vi "Build Full Item List.vi"(11 "Components":T2[](array[typedef])) -> (3 "Total Ingredients":T1[](array[typedef]))   [LabVIEW 2020, in "App.lvclass"]
uses:
  App.lvclass
  Blueprint Qty.ctl
  Blueprint/Blueprint.lvclass
  C:/dev/LabVIEW/Good Company Calc/Item/Item.lvclass
  Item/Ingredient.ctl
  Item/Item.lvclass
  Item Batch.ctl
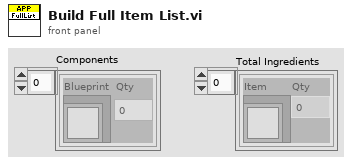
[diagram p1: front panel]
types:
  T1 = typedef "Item.lvclass/Ingredient.ctl" = cluster{"Item":refnum<class "Item.lvclass">, "Qty":dbl}
  T2 = typedef "App.lvclass/Blueprint Qty.ctl" = cluster{"Blueprint":refnum<class "Blueprint.lvclass">, "Qty":dbl}
  T3 = typedef "App.lvclass/Item Batch.ctl" = cluster{"Qty Needed":dbl, "Qty per Batch":dbl, "Batches":dbl}
  T4 = typedef "Item.lvclass/Craft Station.ctl" = cluster{"Station":refnum<class "Workstation.lvclass">, "Craft Time":dbl, "Qty Made":dbl}
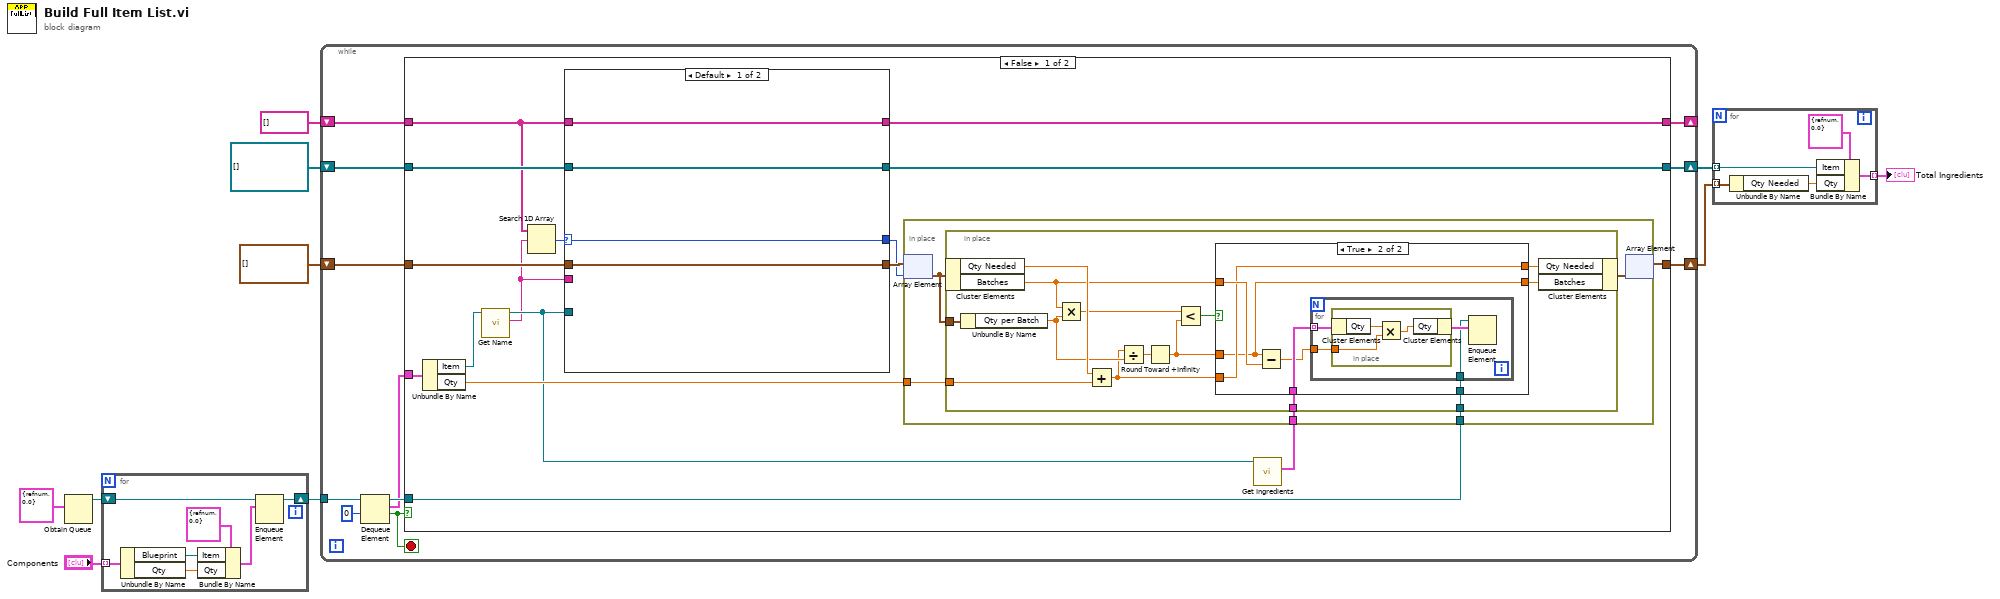
[diagram p0: block diagram]
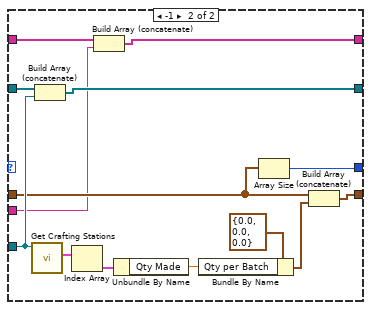
[diagram p2: hidden frame]
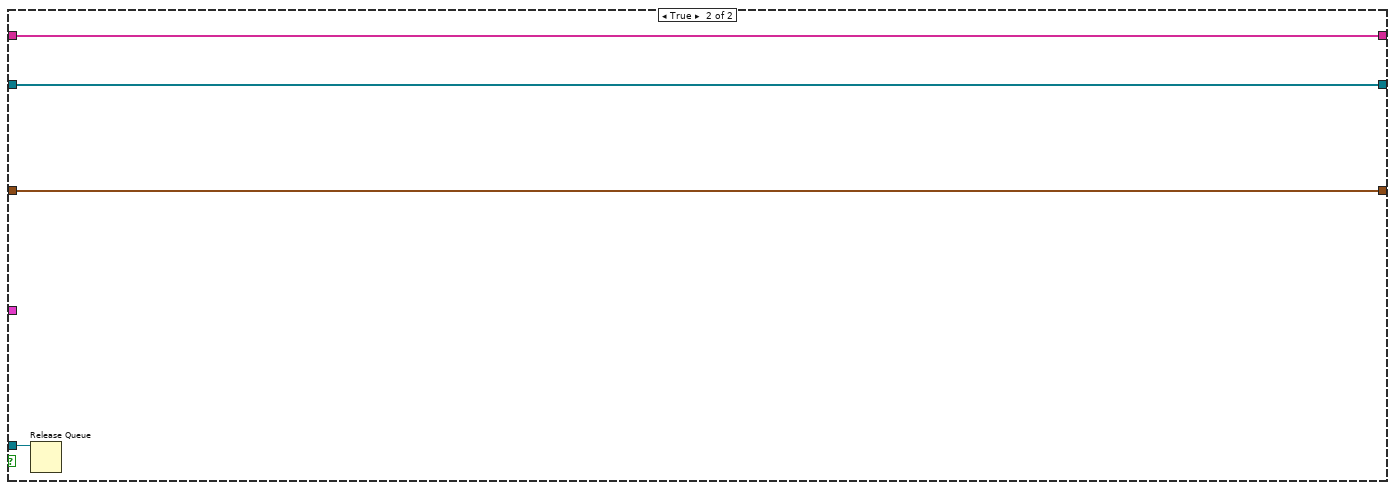
[diagram p4: hidden frame]
diagram:
  n1 = Obtain Queue(element data type=T1 {"Item"=refnum, "Qty"=0.0} ("Ingredient")) -> (queue out=w9:refnum<queue>)  [unwired: 4 in, 2 out]
  n2 = for {
    shift-right: [w16] -> w7
    shift-left: w9 -> [w17]
    tunnel: "Components" -> [w15] mode=indexing
    n3 = Unbundle By Name(w15) -> ("Blueprint"=w13:refnum<class "Blueprint.lvclass">, "Qty"=w12:dbl)
    n4 = Bundle By Name(cluster=T1 {"Item"=refnum, "Qty"=0.0} ("Ingredient"), "Item"=w13, "Qty"=w12) -> (w11:T1)
    n5 = Enqueue Element(queue=w17, element=w11) -> (queue out=w16:refnum<queue>)  [unwired: 2 in, 2 out]
  }
  n6 = while {
    shift-right: [w20] -> w2
    shift-left: T3[] [] -> [w21]
    shift-right: [w22] -> w4
    shift-left: refnum<class "Item.lvclass">[] [] -> [w23]
    tunnel: w7 -> [w28]
    shift-right: [w18] -> _
    shift-left: string[] [] -> [w19]
    stop <- w26 stop-if-true
    n7 = Dequeue Element(queue=w28, timeout in ms (-1)=0) -> (queue out=w25:refnum<queue>, element=w24:T1, timed out?=w26:bool)  [unwired: 1 in, 1 out]
    n8 = case shown="False" w26 {
      tunnel: w25 -> [w39 w99]
      tunnel: w24 -> [w44 _]
      tunnel: w23 -> [w37 w100]
      tunnel: [w43 w100] -> w22
      tunnel: w21 -> [w36 w98]
      tunnel: [w42 w98] -> w20
      tunnel: w19 -> [w32 w97]
      tunnel: [w29 w97] -> w18
      frame False {
        n9 = Unbundle By Name(w44) -> ("Item"=w33:refnum<class "Item.lvclass">, "Qty"=w41:dbl)
        n10 = call-dynamic "Get Name.vi"("Item in"=w33) -> ("Name"=w30:string, "Item out"=w31:refnum<class "Item.lvclass">)  [unwired: 8 in, 1 out]
        n11 = Search 1D Array(1D array=w32, element=w30) -> (index of element=w38:i32)  [unwired: 1 in]
        n12 = case shown="Default" w38 {
          selector: w38 -> [w46 _]
          tunnel: w37 -> [w48 w56]
          tunnel: w31 -> [_ w55]
          tunnel: w36 -> [w47 w53]
          tunnel: [w48 w54] -> w43
          tunnel: [w47 w57] -> w35
          tunnel: [w46 w52] -> w34
          tunnel: w32 -> [w45 w51]
          tunnel: w30 -> [_ w50]
          tunnel: [w45 w49] -> w29
          frame Default {
          }
          frame -1 {
            n13 = call-dynamic "Get Crafting Stations.vi"("Item in"=w55) -> ("Stations"=w62:T4[])  [unwired: 8 in, 2 out]
            n14 = Build Array (concatenate)(w56, w55) -> (w54:refnum<class "Item.lvclass">[])
            n15 = Index Array(array=w62) -> (element=w61:T4)  [unwired: 1 in]
            n16 = Build Array (concatenate)(w51, w50) -> (w49:string[])
            n17 = Unbundle By Name(w61) -> ("Qty Made"=w59:dbl)
            n18 = Bundle By Name(cluster=T3 {"Qty Needed"=0.0, "Qty per Batch"=0.0, "Batches"=0.0} ("Item Batch"), "Qty per Batch"=w59) -> (w58:T3)
            n19 = Array Size(array=w53) -> (size(s)=w52:i32)
            n20 = Build Array (concatenate)(w53, w58) -> (w57:T3[])
          }
        }
        n21 = call-dynamic "Get Ingredients.vi"("Item in"=w31) -> ("Ingredients"=w40:T1[])  [unwired: 8 in, 2 out]
        n22 = in-place {
          in-place-border: w41 -> [w67]
          in-place-border: w40 -> [w64]
          in-place-border: w39 -> [w63]
          n23 = in-place-array #1(w35, w34) -> (w65:T3)
          n24 = in-place {
            in-place-border: w67 -> [w81]
            in-place-border: w65 -> [w79]
            in-place-border: w64 -> [w69]
            in-place-border: w63 -> [w68]
            n25 = in-place-cluster #2(w65) -> ("Qty Needed"=w80:dbl, "Batches"=w74:dbl)
            n26 = Unbundle By Name(w79) -> ("Qty per Batch"=w78:dbl)
            n27 = Multiply(x=w74, y=w78) -> (x*y=w76:dbl)
            n28 = Add(x=w80, y=w81) -> (x+y=w75:dbl)
            n29 = Divide(x=w75, y=w78) -> (x/y=w77:dbl)
            n30 = Round Toward +Infinity(x=w77) -> (ceil(x): smallest int >= x=w72:dbl)
            n31 = Less?(x=w76, y=w72) -> (x < y?=w73:bool)
            n32 = case shown="True" w73 {
              tunnel: w75 -> [w82 w88]
              tunnel: w74 -> [w83 w89]
              tunnel: w72 -> [_ w87]
              tunnel: [w82 w88] -> w71
              tunnel: [w83 w87] -> w70
              tunnel: w69 -> [_ w86]
              tunnel: w68 -> [_ w84]
              frame False {
              }
              frame True {
                n33 = Subtract(x=w87, y=w89) -> (x-y=w85:dbl)
                n34 = for {
                  tunnel: w86 -> [w90] mode=indexing
                  tunnel: w85 -> [w92]
                  tunnel: w84 -> [w91]
                  n35 = in-place {
                    in-place-border: w92 -> [w95]
                    n36 = in-place-cluster #3(w90) -> ("Qty"=w96:dbl)
                    n37 = Multiply(x=w96, y=w95) -> (x*y=w94:dbl)
                    n38 = in-place-cluster #3("Qty"=w94) -> (w93:T1)
                  }
                  n39 = Enqueue Element(queue=w91, element=w93) -> ()  [unwired: 2 in, 3 out]
                }
              }
            }
            n40 = in-place-cluster #2("Qty Needed"=w71, "Batches"=w70) -> (w66:T3)
          }
          n41 = in-place-array #1(w66) -> (w42:T3[])  [unwired: 1 out]
        }
      }
      frame True {
        n42 = Release Queue(queue=w99) -> ()  [unwired: 2 in, 3 out]
      }
    }
  }
  n43 = for {
    tunnel: w4 -> [w104] mode=indexing
    tunnel: [w103] -> w3 mode=indexing
    tunnel: w2 -> [w102] mode=indexing
    n44 = Unbundle By Name(w102) -> ("Qty Needed"=w101:dbl)
    n45 = Bundle By Name(cluster=T1 {"Item"=refnum, "Qty"=0.0} ("Ingredient"), "Item"=w104, "Qty"=w101) -> (w103:T1)
  }
  "Total Ingredients" <- w3
